vi "power read sim.vi"(7 "Max Voltage in (V)":dbl=8.5 format="%.2f", 11 "error in (no error)":errorcluster) -> (8 "normalized Power Read (0-1)":dbl=0.0244140625 format="%.2f", 15 "error out":errorcluster)   [LabVIEW 2016]
doc: "This one shot VI reads the power using the thermal simulator\n\nPaul K Dixon\nPhysics 350\nPaul K Dixon"
uses:
  therm sim/therm sim kernel/globals/therm sim globals.vi
panel:
  in  "channel (0)":tag="Dev1/ai0"
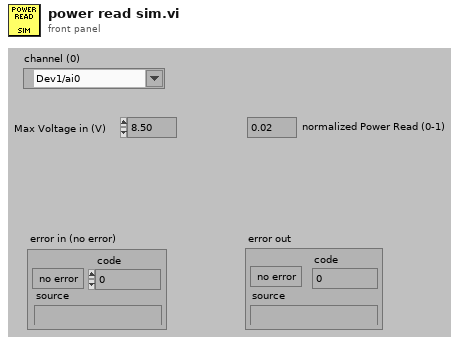
[diagram p1: front panel]
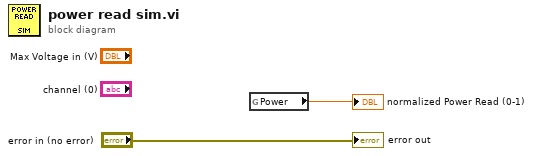
[diagram p0: block diagram]
diagram:
  n1 = global read "therm sim globals.vi" "Power"() -> (→"normalized Power Read (0-1)":dbl)
  "error out" <- "error in (no error)"
